vi "Stop Acquisition.vi"(8 "error in (no error)":errorcluster, 11 "DAQmx in":refnum<class "DAQmx.lvclass">) -> (0 "error out":errorcluster, 3 "DAQmx out":refnum<class "DAQmx.lvclass">)   [LabVIEW 2019, in "DAQmx.lvclass"]
uses:
  DAQmx.lvclass
  DAQmx.lvclass/DAQmx.ctl
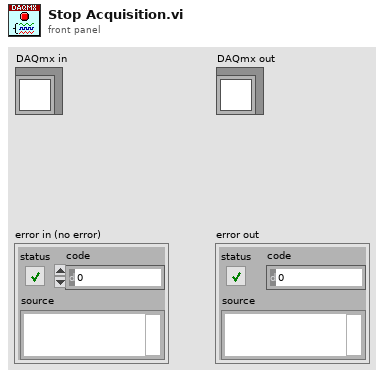
[diagram p1: front panel]
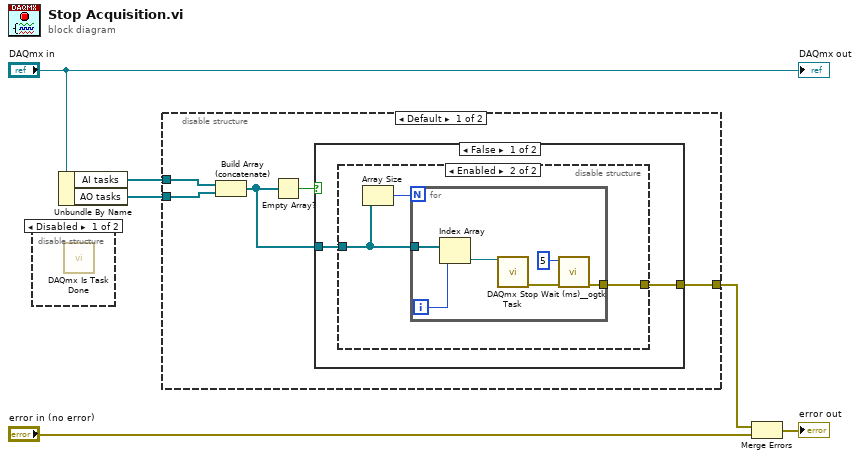
[diagram p0: block diagram]
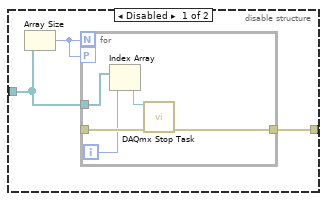
[diagram p3: hidden frame]
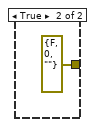
[diagram p4: hidden frame]
diagram:
  n1 = disable-structure shown="Disabled" {
    frame Disabled {
      n2 = call <vilib>:"DAQmx Is Task Done.vi"() -> ()  [unwired: 13 in, 3 out]
    }
    frame Enabled {
    }
  }
  n3 = Unbundle By Name("DAQmx in") -> ("AI tasks"=w5:refnum<k21>[], "AO tasks"=w6:refnum<k21>[])
  n4 = disable-structure shown="Default" {
    disable-tunnel: [w9 _] -> w2
    disable-tunnel: w6 -> [w10 _]
    disable-tunnel: w5 -> [w11 _]
    frame condition #0 (active) {
      n5 = Build Array (concatenate)(w11, w10) -> (w7:refnum<k21>[])
      n6 = Empty Array?(array=w7) -> (empty?=w8:bool)
      n7 = case shown="False" w8 {
        tunnel: w7 -> [w12 _]
        tunnel: [w13 errorcluster {"status"=FALSE, "code"=0, "source"=""} ("error out")] -> w9
        frame False {
          n8 = disable-structure shown="Enabled" {
            disable-tunnel: [w16 w25] -> w13
            disable-tunnel: w12 -> [w15 w24]
            frame Disabled {
              n9 = Array Size(array=w15) -> (size(s)=w14:i32)
              n10 = for {
                N: w14 -> [_]
                tunnel: w15 -> [w20]
                tunnel: [w22] -> w17
                tunnel: [w21] -> w16
                workers-P: w14 -> [_]
                i -> [w19]
                n11 = Index Array(array=w20, index=w19) -> (element=w18:refnum<k21>)
                n12 = call <vilib>:"DAQmx Stop Task.vi"("task/channels in"=w18, "error in"=w22) -> ("error out"=w21:errorcluster)  [unwired: 12 in, 1 out]
              }
            }
            frame Enabled {
              n13 = Array Size(array=w24) -> (size(s)=w23:i32)
              n14 = for {
                N: w23 -> [_]
                tunnel: w24 -> [w30]
                tunnel: [w27] -> w25
                i -> [w29]
                n15 = Index Array(array=w30, index=w29) -> (element=w28:refnum<k21>)
                n16 = call <vilib>:"DAQmx Stop Task.vi"("task/channels in"=w28) -> ("error out"=w31:errorcluster)  [unwired: 13 in, 1 out]
                n17 = call <userlib>:"Wait (ms)__ogtk.vi"("error in (no error)"=w31, "milliseconds to wait"=u32 5) -> ("error out"=w27:errorcluster)  [unwired: 8 in, 1 out]
              }
            }
          }
        }
        frame True {
        }
      }
    }
    frame condition #1 {
    }
  }
  n18 = Merge Errors(w2, "error in (no error)") -> (→"error out":errorcluster)
  "DAQmx out" <- "DAQmx in"
